vi "Plot Dot.vi"(1 "Diameter":dbl=25.0, 2 "Y":dbl, 3 "X":dbl) -> (0 "Cluster":cluster{dbl, dbl, dbl, dbl})   [LabVIEW 2012]
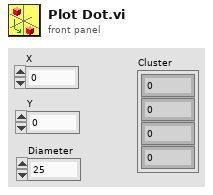
[diagram p1: front panel]
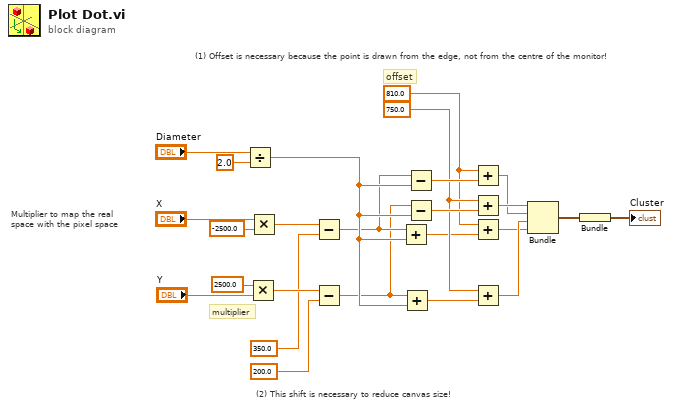
[diagram p0: block diagram]
diagram:
  w12 = 750.0 ("ID")
  w11 = 810.0 ("ID")
  # "Multiplier to map the real \nspace with the pixel space"
  # "(2) This shift is necessary to reduce canvas size!"
  # "(1) Offset is necessary because the point is drawn from the edge, not from the centre of the monitor!"
  # "multiplier"
  # "offset"
  n1 = Divide(x="Diameter", y=2.0) -> (x/y=w8:dbl)
  n2 = Multiply(x=2500.0 ("y"), y="Y") -> (x*y=w3:dbl)
  n3 = Multiply(x="X", y=-2500.0) -> (x*y=w5:dbl)
  n4 = Subtract(x=w5, y=350.0) -> (x-y=w6:dbl)
  n5 = Subtract(x=w3, y=200.0) -> (x-y=w4:dbl)
  n6 = Add(x=w6, y=w8) -> (x+y=w10:dbl)
  n7 = Add(x=w4, y=w8) -> (x+y=w9:dbl)
  n8 = Subtract(x=w6, y=w8) -> (x-y=w19:dbl)
  n9 = Subtract(x=w4, y=w8) -> (x-y=w18:dbl)
  n10 = Add(x=w11, y=w19) -> (x+y=w16:dbl)
  n11 = Add(x=w12, y=w18) -> (x+y=w17:dbl)
  n12 = Add(x=w11, y=w10) -> (x+y=w14:dbl)
  n13 = Add(x=w12, y=w9) -> (x+y=w15:dbl)
  n14 = Bundle(w17, w16, w15, w14) -> (w24:cluster{dbl, dbl, dbl, dbl})  [unwired: 1 in]
  "Cluster" <- w24
  n15 = Bundle(w24) -> ()  [unwired: 1 in, 1 out]
